vi "Control_demo.vi"(1 "stop":bool) -> (7 "liveview":dbl[][](graph))   [LabVIEW 2016]
uses:
  Vital supporting file for labview program/LV-EDSDK-Distribution_0.2/Distribution/EDSDK-Labview.llb/kEdsProperties.ctl
  Vital supporting file for labview program/LV-EDSDK-Distribution_0.2/Distribution/EDSDK-Labview.llb/kEdsCameraCommands.ctl
  Vital supporting file for labview program/C++/Dll for liveview/x64/Debug/Dll for liveview.dll
panel:
  in  "y 4":i16
  in  "y 3":i16
  in  "y 2":i16
  in  "y":i16
  in  "X":cluster{i32, i32}(slide)={0, 24101949} scale=0.0..1000.0
  out "new picture":picture
  in  "Zoom Factor":dbl=0.15
  in  "file name":string="m200test.bmp"
  in  "Path":path=path "C:/Users/Administrator/Desktop"
  out "saved image":picture
  out "output array 2":u32[][](array[numeric])
  out "error out":errorcluster
  in  "shutter":bool
  in  "Shutter speed":u16(ring) items=["1/8000"=160, "1/6400"=157, "1/6000"=156, "1/5000"=155, "1/4000"=152, "1/3200"=149, "1/3000"=148, "1/2500"=147, "1/2000"=144, "1/1600"=141, "1/1500"=140, "1/1250"=139, "1/100"=136, "1/800"=133, "1/640"=131, "1/500"=128, "1/400"=125, "1/320"=123, "1/250"=120, "1/200"=117, "1/160"=115, "1/125"=112, "1/100"=109, "1/80"=107, "1/60"=104, "1/50"=101, "1/40"=99, "1/30"=96, "1/25"=93, "1/8"=80, "1/6"=77, "1/5"=75, "1/4"=72, "0\"3"=69, "0\"4"=67, "0\"5"=64, "0\"6"=61, "0\"7"=60, "0\"8"=59, "1\""=56, "1\"3"=53, "1\"5"=52, "1\"6"=51, "2\""=48, "2\"5"=45, "3\""=44, "3\"2"=43, "4\""=40, "5\""=37, "6\""=35, "8\""=32, "10\""=29, "13\""=27, "15\""=24, "20\""=21, "25\""=19, "30\""=16]
  in  "ISO":u32(ring) items=["Auto"=0, "50"=64, "100"=72, "125"=75, "160"=77, "200"=80, "250"=83, "320"=85, "400"=88, "500"=91, "640"=93, "800"=96, "1000"=99, "1250"=101, "1600"=104, "2000"=107, "2500"=109, "3200"=112, "4000"=115, "5000"=117, "6400"=120, "8000"=123, "10000"=125, "12800"=128, "25600"=136, "51200"=144, "102400"=152, "204800"=160, "409600"=168]
  out "outDeviceInfo":T1
  in  "error in (no error)":errorcluster
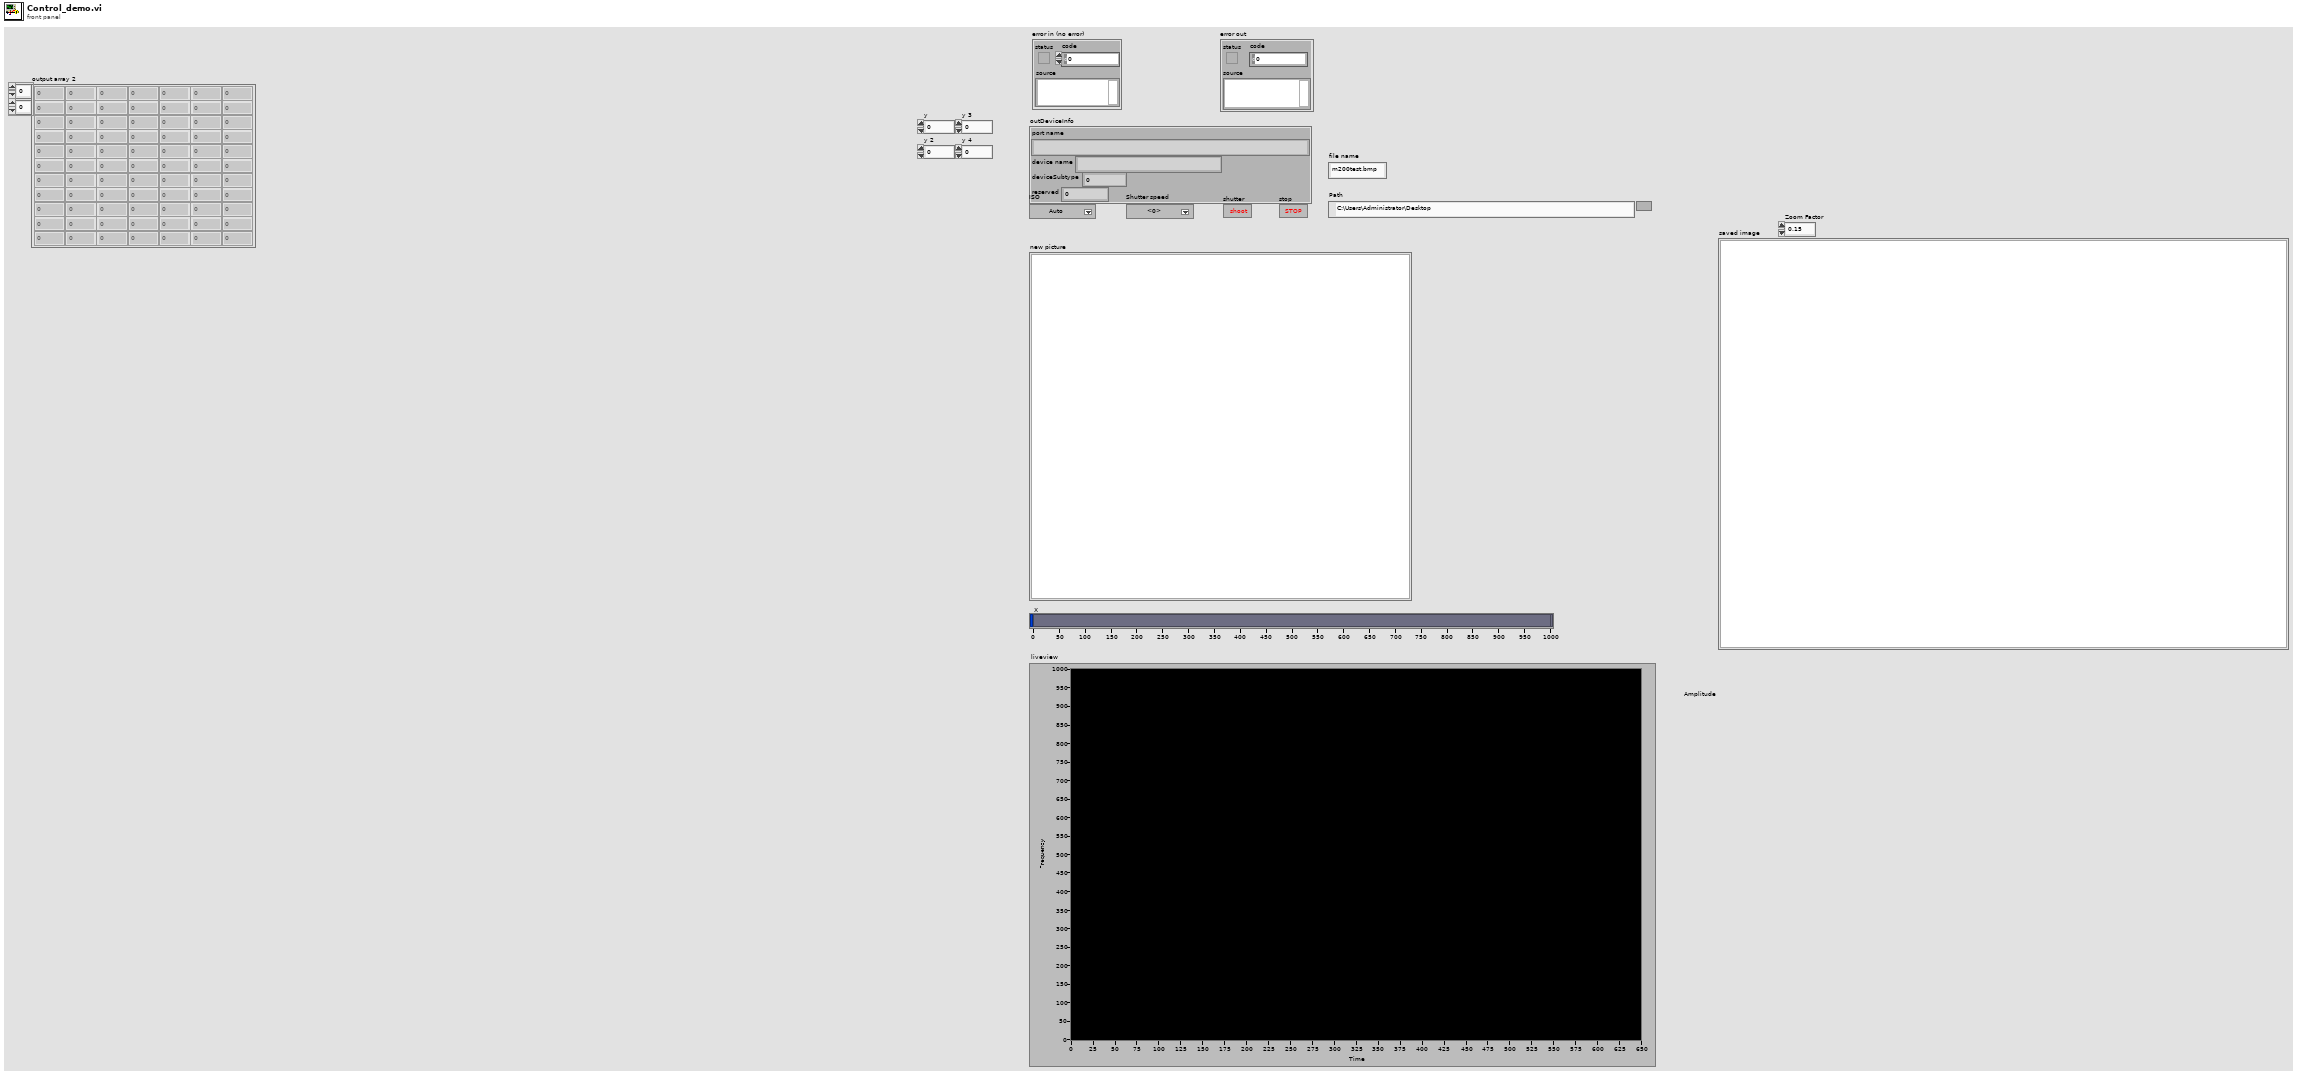
[diagram p1: front panel]
types:
  T1 = cluster{"port name":string, "device name":string, "deviceSubtype":u32, "reserved":u32}
  T2 = typedef "kEdsProperties.ctl" = u32
  T3 = enum16{"open", "replace", "create", "open or create", "replace or create", "replace or create with confirmation"}
  T4 = cluster{"Width":u16, "Style":enum32{"Solid", "Dash", "Dot", "DashDot", "DashDotDot"}}
  T5 = typedef "LVBoundsTypeDef.ctl" = cluster{"Width":u32, "Height":u32}
  T6 = typedef "imagedata.ctl" = cluster{"image type":i32, "image depth":i32, "image":u8[], "mask":u8[], "colors":u32[], "Rectangle":cluster{"left":i16, "top":i16, "right":i16, "bottom":i16}}
  T7 = cluster{"left":i16, "top":i16, "right":i16, "bottom":i16}
  T8 = typedef "kEdsCameraCommands.ctl" = u32
  T9 = typedef "LVMouseTypeDef.ctl" = cluster{"Mouse Position":cluster{"X":i32, "Y":i32}, "Mouse Modifiers":cluster{"Button Down":bool, "Shift Mod":bool, "Menu Mod":bool, "Option Mod":bool}}
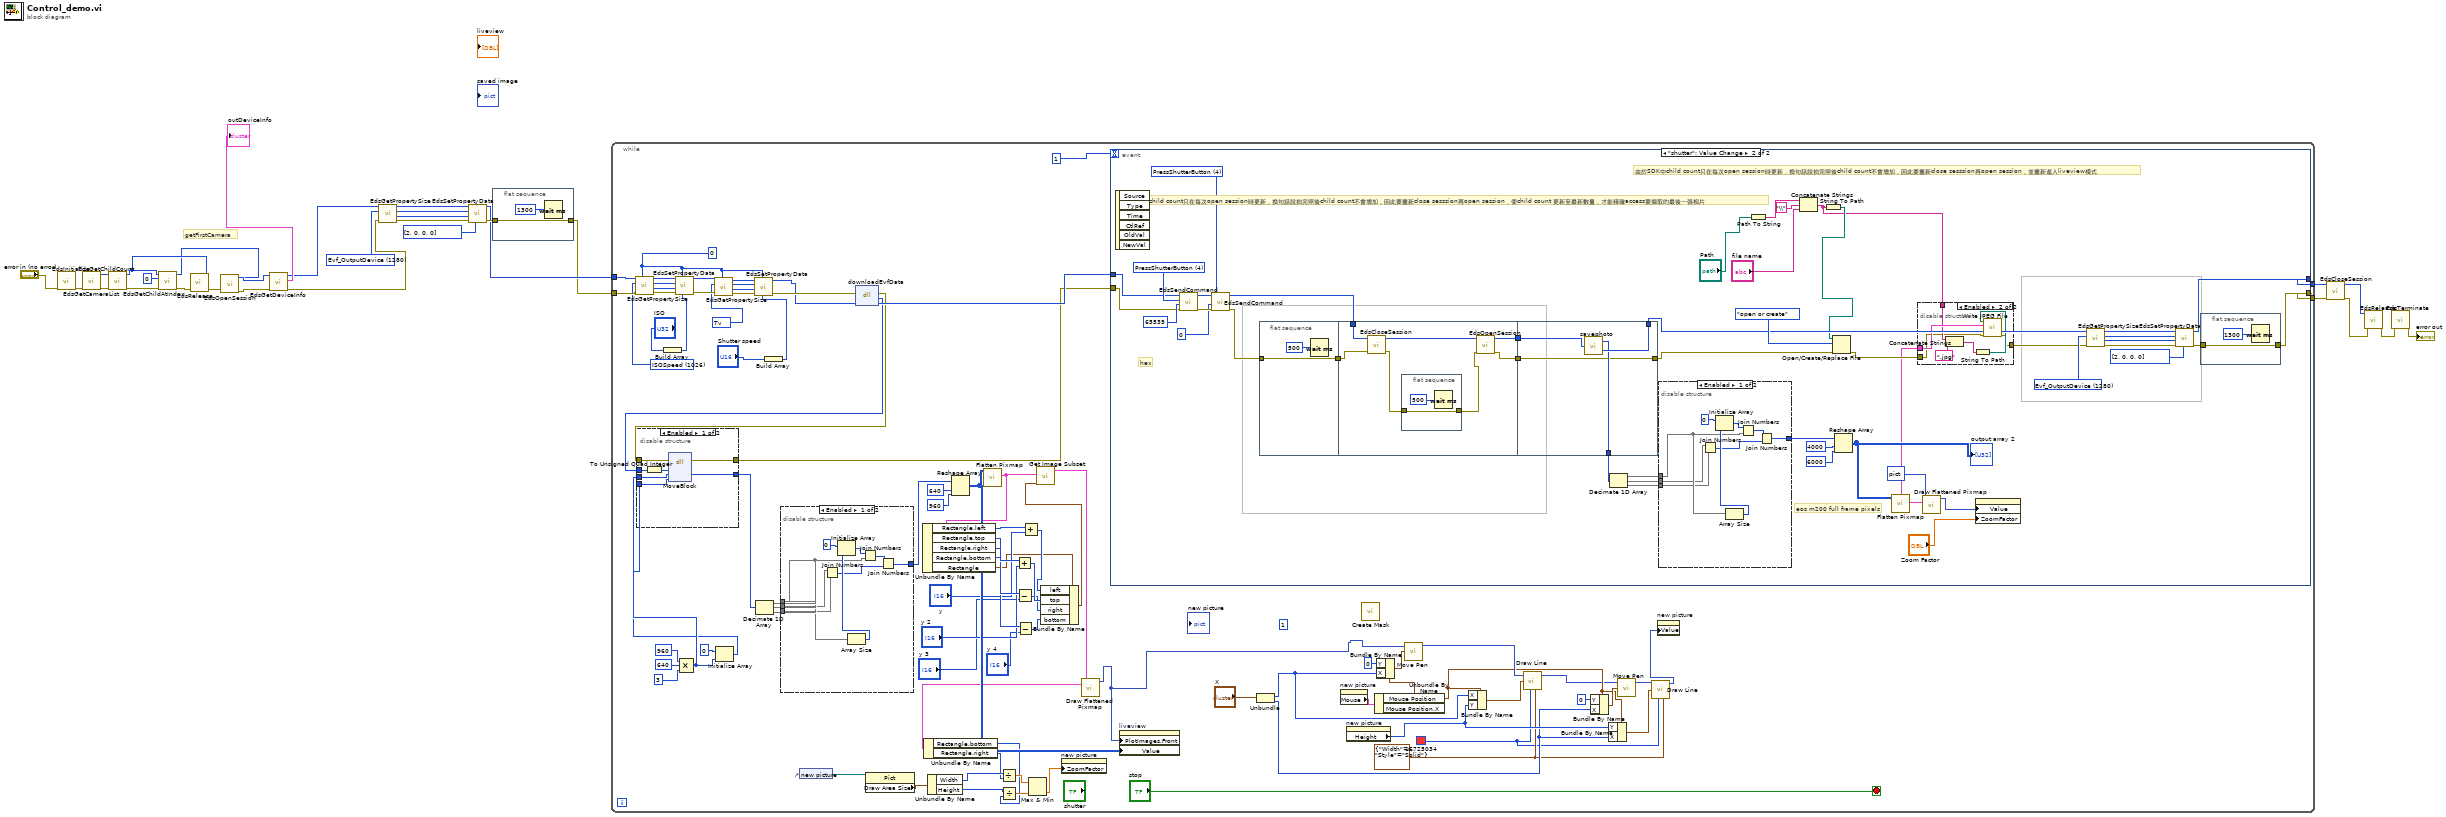
[diagram p0: block diagram]
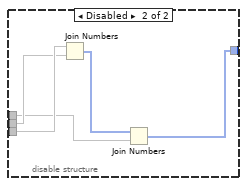
[diagram p2: hidden frame]
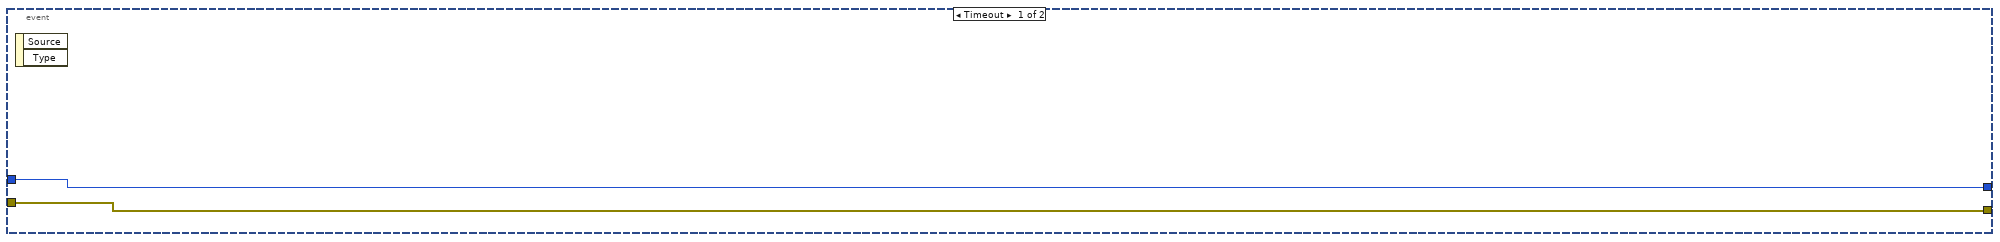
[diagram p4: hidden frame]
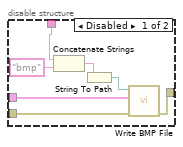
[diagram p5: hidden frame]
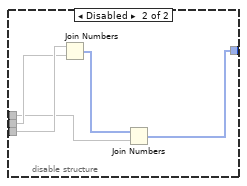
[diagram p6: hidden frame]
diagram:
  w5 = T2 1280 items=["Unknown"=65535, "ProductName"=2, "BodyID"=3, "OwnerName"=4, "MakerName"=5, "DateTime"=6, "FirmwareVersion"=7, "BatteryLevel"=8, "CFn"=9, "SaveTo"=11, "CurrentStorage"=12, "CurrentFolder"=13, "MyMenu"=14, "BatteryQuality"=16, "HDDirectoryStructure"=32, "ImageQuality"=256, "JpegQuality"=257, "Orientation"=258, "ICCProfile"=259, "FocusInfo"=260, "DigitalExposure"=261, "WhiteBalance"=262, "ColorTemperature"=263, "WhiteBalanceShift"=264, "Contrast"=265, "ColorSaturation"=266, "ColorTone"=267, "Sharpness"=268, "ColorSpace"=269, "ToneCurve"=270, "PhotoEffect"=271, "FilterEffect"=272, "ToningEffect"=273, "ParameterSet"=274, "ColorMatrix"=275, "PictureStyle"=276, "PictureStyleDesc"=277, "ETTL2Mode"=279, "PictureStyleCaption"=512, "Linear"=768, "ClickWBPoint"=769, "WBCoeffs"=770, "GPSVersionID"=2048, "GPSLatitudeRef"=2049, "GPSLatitude"=2050, "GPSLongitudeRef"=2051, "GPSLongitude"=2052, "GPSAltitudeRef"=2053, "GPSAltitude"=2054, "GPSTimeStamp"=2055, "GPSSatellites"=2056, "GPSStatus"=2057, "GPSMapDatum"=2066, "GPSDateStamp"=2077, "AtCapture_Flag"=2147483648, "AEMode"=1024, "DriveMode"=1025, "ISOSpeed"=1026, "MeteringMode"=1027, "AFMode"=1028, "Av"=1029, "Tv"=1030, "ExposureCompensation"=1031, "FlashCompensation"=1032, "FocalLength"=1033, "AvailableShots"=1034, "Bracket"=1035, "WhiteBalanceBracket"=1036, "LensName"=1037, "AEBracket"=1038, "FEBracket"=1039, "ISOBracket"=1040, "NoiseReduction"=1041, "FlashOn"=1042, "RedEye"=1043, "FlashMode"=1044, "LensStatus"=1046, "Artist"=1048, "Copyright"=1049, "DepthOfField"=1051, "EFCompensation"=1054, "Evf_OutputDevice"=1280, "Evf_Mode"=1281, "Evf_WhiteBalance"=1282, "Evf_ColorTemperature"=1283, "Evf_DepthOfFieldPreview"=1284, "Evf_Zoom"=1287, "Evf_ZoomPosition"=1288, "Evf_FocusAid"=1289, "Evf_Histogram"=1290, "Evf_ImagePosition"=1291, "Evf_HistogramStatus"=1292, "Evf_AFMode"=1294, "Evf_CoordinateSystem"=1344, "Evf_ZoomRect"=1345] ("inPropertyID")
  # "getFirstCamera"
  n1 = call "EdsInitialize.vi"("error in (no error)"="error in (no error)") -> ("error out"=w29:errorcluster)  [unwired: 10 in]
  n2 = call "EdsGetCameraList.vi"("error in"=w29) -> ("error out"=w28:errorcluster, "outCameraListRef"=w24:u32)  [unwired: 9 in]
  n3 = call "EdsGetChildCount.vi"("error in"=w28, "inRef"=w24) -> ("error out"=w27:errorcluster, "inRef dup"=w23:u32)  [unwired: 7 in, 1 out]
  n4 = call "EdsGetChildAtIndex.vi"("error in"=w27, "index"=u32 0, "inRef"=w23) -> ("error out"=w25:errorcluster, "outRef"=w19:u32)  [unwired: 7 in]
  n5 = call "EdsRelease.vi"("error in"=w25, "inRef"=w23) -> ("error out"=w22:errorcluster)  [unwired: 7 in, 2 out]
  n6 = call "EdsOpenSession.vi"("error in"=w22, "inCameraRef"=w19) -> ("error out"=w20:errorcluster, "inCameraRef dup"=w21:u32)  [unwired: 8 in]
  n7 = call "EdsGetDeviceInfo.vi"("error in"=w20, "inCameraRef"=w21) -> ("error out"=w2:errorcluster, "outDeviceInfo"=→"outDeviceInfo":T1, "inCameraRef dup"=w4:u32)  [unwired: 7 in]
  n8 = call "EdsGetPropertySize.vi"("error in"=w2, "inPropertyID"=w5, "inRef"=w4) -> ("error out"=w8:errorcluster, "outSize"=w9:u32, "inPropertyID dup"=w7:T2, "inRef dup"=w6:u32)  [unwired: 4 in, 1 out]
  n9 = call "EdsSetPropertyData.vi"("inPropertyData"=u8[] [2, 0, 0, 0], "error in"=w8, "inPropertySize"=w9, "inPropertyID"=w7, "inRef"=w6) -> ("error out"=w11:errorcluster, "inRef dup"=w3:u32)  [unwired: 5 in]
  n10 = flat-sequence {
    tunnel: w11 -> [w32]
    tunnel: [w32] -> w1
    frame #0 {
      n11 = Wait (ms)(milliseconds to wait=u32 1300) -> ()  [unwired: 1 out]
    }
  }
  n12 = while {
    tunnel: w3 -> [w100]
    tunnel: w1 -> [w119]
    tunnel: [w78] -> w13
    tunnel: [w79] -> w12
    stop <- "stop" stop-if-true
    w52 = T4 {"Width"=6, "Style"=enum."Solid"} ("pen")
    w51 = u32 16725034 ("color(black)")
    (unwired) 1
    w101 = T2 1030 items=["Unknown"=65535, "ProductName"=2, "BodyID"=3, "OwnerName"=4, "MakerName"=5, "DateTime"=6, "FirmwareVersion"=7, "BatteryLevel"=8, "CFn"=9, "SaveTo"=11, "CurrentStorage"=12, "CurrentFolder"=13, "MyMenu"=14, "BatteryQuality"=16, "HDDirectoryStructure"=32, "ImageQuality"=256, "JpegQuality"=257, "Orientation"=258, "ICCProfile"=259, "FocusInfo"=260, "DigitalExposure"=261, "WhiteBalance"=262, "ColorTemperature"=263, "WhiteBalanceShift"=264, "Contrast"=265, "ColorSaturation"=266, "ColorTone"=267, "Sharpness"=268, "ColorSpace"=269, "ToneCurve"=270, "PhotoEffect"=271, "FilterEffect"=272, "ToningEffect"=273, "ParameterSet"=274, "ColorMatrix"=275, "PictureStyle"=276, "PictureStyleDesc"=277, "ETTL2Mode"=279, "PictureStyleCaption"=512, "Linear"=768, "ClickWBPoint"=769, "WBCoeffs"=770, "GPSVersionID"=2048, "GPSLatitudeRef"=2049, "GPSLatitude"=2050, "GPSLongitudeRef"=2051, "GPSLongitude"=2052, "GPSAltitudeRef"=2053, "GPSAltitude"=2054, "GPSTimeStamp"=2055, "GPSSatellites"=2056, "GPSStatus"=2057, "GPSMapDatum"=2066, "GPSDateStamp"=2077, "AtCapture_Flag"=2147483648, "AEMode"=1024, "DriveMode"=1025, "ISOSpeed"=1026, "MeteringMode"=1027, "AFMode"=1028, "Av"=1029, "Tv"=1030, "ExposureCompensation"=1031, "FlashCompensation"=1032, "FocalLength"=1033, "AvailableShots"=1034, "Bracket"=1035, "WhiteBalanceBracket"=1036, "LensName"=1037, "AEBracket"=1038, "FEBracket"=1039, "ISOBracket"=1040, "NoiseReduction"=1041, "FlashOn"=1042, "RedEye"=1043, "FlashMode"=1044, "LensStatus"=1046, "Artist"=1048, "Copyright"=1049, "DepthOfField"=1051, "EFCompensation"=1054, "Evf_OutputDevice"=1280, "Evf_Mode"=1281, "Evf_WhiteBalance"=1282, "Evf_ColorTemperature"=1283, "Evf_DepthOfFieldPreview"=1284, "Evf_Zoom"=1287, "Evf_ZoomPosition"=1288, "Evf_FocusAid"=1289, "Evf_Histogram"=1290, "Evf_ImagePosition"=1291, "Evf_HistogramStatus"=1292, "Evf_AFMode"=1294, "Evf_CoordinateSystem"=1344, "Evf_ZoomRect"=1345] ("inPropertyID")
    w103 = 0 ("inParam")
    w113 = T2 1026 items=["Unknown"=65535, "ProductName"=2, "BodyID"=3, "OwnerName"=4, "MakerName"=5, "DateTime"=6, "FirmwareVersion"=7, "BatteryLevel"=8, "CFn"=9, "SaveTo"=11, "CurrentStorage"=12, "CurrentFolder"=13, "MyMenu"=14, "BatteryQuality"=16, "HDDirectoryStructure"=32, "ImageQuality"=256, "JpegQuality"=257, "Orientation"=258, "ICCProfile"=259, "FocusInfo"=260, "DigitalExposure"=261, "WhiteBalance"=262, "ColorTemperature"=263, "WhiteBalanceShift"=264, "Contrast"=265, "ColorSaturation"=266, "ColorTone"=267, "Sharpness"=268, "ColorSpace"=269, "ToneCurve"=270, "PhotoEffect"=271, "FilterEffect"=272, "ToningEffect"=273, "ParameterSet"=274, "ColorMatrix"=275, "PictureStyle"=276, "PictureStyleDesc"=277, "ETTL2Mode"=279, "PictureStyleCaption"=512, "Linear"=768, "ClickWBPoint"=769, "WBCoeffs"=770, "GPSVersionID"=2048, "GPSLatitudeRef"=2049, "GPSLatitude"=2050, "GPSLongitudeRef"=2051, "GPSLongitude"=2052, "GPSAltitudeRef"=2053, "GPSAltitude"=2054, "GPSTimeStamp"=2055, "GPSSatellites"=2056, "GPSStatus"=2057, "GPSMapDatum"=2066, "GPSDateStamp"=2077, "AtCapture_Flag"=2147483648, "AEMode"=1024, "DriveMode"=1025, "ISOSpeed"=1026, "MeteringMode"=1027, "AFMode"=1028, "Av"=1029, "Tv"=1030, "ExposureCompensation"=1031, "FlashCompensation"=1032, "FocalLength"=1033, "AvailableShots"=1034, "Bracket"=1035, "WhiteBalanceBracket"=1036, "LensName"=1037, "AEBracket"=1038, "FEBracket"=1039, "ISOBracket"=1040, "NoiseReduction"=1041, "FlashOn"=1042, "RedEye"=1043, "FlashMode"=1044, "LensStatus"=1046, "Artist"=1048, "Copyright"=1049, "DepthOfField"=1051, "EFCompensation"=1054, "Evf_OutputDevice"=1280, "Evf_Mode"=1281, "Evf_WhiteBalance"=1282, "Evf_ColorTemperature"=1283, "Evf_DepthOfFieldPreview"=1284, "Evf_Zoom"=1287, "Evf_ZoomPosition"=1288, "Evf_FocusAid"=1289, "Evf_Histogram"=1290, "Evf_ImagePosition"=1291, "Evf_HistogramStatus"=1292, "Evf_AFMode"=1294, "Evf_CoordinateSystem"=1344, "Evf_ZoomRect"=1345] ("inPropertyID")
    n13 = call "EdsGetPropertySize.vi"("inParam"=w103, "error in"=w119, "inPropertyID"=w113, "inRef"=w100) -> ("error out"=w115:errorcluster, "outSize"=w114:u32, "inPropertyID dup"=w116:T2, "inRef dup"=w117:u32)  [unwired: 3 in, 1 out]
    n14 = Build Array("ISO") -> (w111:u32[])
    n15 = call "EdsSetPropertyData.vi"("inPropertyData"=w111, "inParam"=w103, "error in"=w115, "inPropertySize"=w114, "inPropertyID"=w116, "inRef"=w117) -> ("error out"=w109:errorcluster, "inRef dup"=w102:u32)  [unwired: 4 in]
    n16 = Compound Arithmetic op=MULTIPLY(960 ("dimension size"), 640 ("dimension size"), 3 ("dimension size")) -> (w89:i32)
    n17 = call "EdsGetPropertySize.vi"("inParam"=w103, "error in"=w109, "inPropertyID"=w101, "inRef"=w102) -> ("error out"=w108:errorcluster, "outSize"=w106:u32, "inPropertyID dup"=w110:T2, "inRef dup"=w107:u32)  [unwired: 3 in, 1 out]
    n18 = Initialize Array ("初始化数组")(u8 0 ("element"), w89) -> (w88:u8[])
    n19 = Build Array("Shutter speed") -> (w104:u16[])
    n20 = call "EdsSetPropertyData.vi"("inPropertyData"=w104, "inParam"=w103, "error in"=w108, "inPropertySize"=w106, "inPropertyID"=w110, "inRef"=w107) -> ("error out"=w99:errorcluster, "inRef dup"=w98:u32)  [unwired: 4 in]
    n21 = control-ref of="new picture"() -> (w68:refnum<vi>)
    n22 = dll-call lib="D:/All users/PoSheng/src/labview for canon om/Vital supporting file for labview program/C++/Dll for liveview/x64/Debug/Dll for liveview.dll" fn="downloadEvfData"(error in=w99, "CamRef"=w98) -> (error out=w83:errorcluster, "return type"=w81:i64, "CamRef"=w97:u32)  [unwired: 2 in, 1 out]
    n23 = disable-structure shown="Enabled" {
      disable-tunnel: [w140 w141] -> w82
      disable-tunnel: w81 -> [w139 _]
      disable-tunnel: w83 -> [w138 w141]
      disable-tunnel: w88 -> [w137 _]
      disable-tunnel: w89 -> [w136 _]
      disable-tunnel: [w134 _] -> w96
      frame Enabled {
        n24 = To Unsigned Quad Integer(1:w139) -> (0:w135:u64)
        n25 = dll-call lib="LabVIEW" fn="MoveBlock"(error in=w138, "src"=w135, "dst"=w137, "size"=w136) -> (error out=w140:errorcluster, "dst"=w134:u8[])  [unwired: 5 in, 1 out]
      }
      frame Disabled {
      }
    }
    n26 = Decimate 1D Array(w96) -> (w91:u8[], w90:u8[], w92:u8[])
    n27 = disable-structure shown="Enabled" {
      disable-tunnel: w90 -> [w121 w130]
      disable-tunnel: w91 -> [w122 w129]
      disable-tunnel: w92 -> [w120 w131]
      disable-tunnel: [w123 w132] -> w93
      frame Enabled {
        n28 = Join Numbers(hi=w121, lo=w120) -> ((hi.lo)=w124:u16[])
        n29 = Array Size(array=w122) -> (size(s)=w127:i32)
        n30 = Initialize Array(u8 0, w127) -> (w126:u8[])
        n31 = Join Numbers(hi=w126, lo=w122) -> ((hi.lo)=w125:u16[])
        n32 = Join Numbers(hi=w125, lo=w124) -> ((hi.lo)=w123:u32[])
      }
      frame Disabled {
        n33 = Join Numbers(hi=w131, lo=w130) -> ((hi.lo)=w133:u16[])
        n34 = Join Numbers(hi=w133, lo=w129) -> ((hi.lo)=w132:u32[])
      }
    }
    n35 = property on="Property Node" class="Pict"(reference=w68) -> ("Draw Area Size"=w76:T5)  [unwired: 1 in, 2 out]
    n36 = Unbundle By Name(w76) -> ("Width"=w75:u32, "Height"=w73:u32)
    n37 = Reshape Array(w93, 640 ("dimension size"), 960 ("dimension size")) -> (w80:u32[][])
    n38 = call <vilib>:"Flatten Pixmap.vi"("24-bit pixmap"=w80) -> ("image data"=w47:T6)  [unwired: 10 in]
    n39 = Unbundle By Name(w47) -> ("Rectangle.left"=w46:i16, "Rectangle.top"=w45:i16, "Rectangle.right"=w44:i16, "Rectangle.bottom"=w43:i16, "Rectangle"=w37:T7)
    n40 = Add(x=w45, y="y 2") -> (x+y=w35:i16)
    n41 = Subtract(x=w44, y="y 3") -> (x-y=w34:i16)
    n42 = Subtract(x=w43, y="y 4") -> (x-y=w33:i16)
    n43 = Add(x=w46, y="y") -> (x+y=w38:i16)
    n44 = Bundle By Name(cluster=w37, "left"=w38, "top"=w35, "right"=w34, "bottom"=w33) -> (w36:T7)
    n45 = call <vilib>:"Get Image Subset.vi"("subset rect"=w36, "image data"=w47) -> ("image subset"=w48:T6)  [unwired: 4 in, 1 out]
    n46 = Unbundle By Name(w48) -> ("Rectangle.bottom"=w70:i16, "Rectangle.right"=w74:i16)
    n47 = Divide(x=w75, y=w74) -> (x/y=w72:dbl)
    n48 = Divide(x=w73, y=w70) -> (x/y=w71:dbl)
    n49 = Max & Min(x=w72, y=w71) -> (min(x,y)=w69:dbl)  [unwired: 1 out]
    n50 = property on="new picture" class="Pict"("ZoomFactor"=w69) -> ()  [unwired: 2 in, 2 out]
    n51 = call <vilib>:"Draw Flattened Pixmap.vi"("image data"=w48) -> ("new picture"=w62:picture)  [unwired: 8 in]
    n52 = event shown="[1] \"shutter\": Value Change" {
      selector: _ -> [_ _]
      dyn-events: _ -> [_ _]
      timeout: 1 -> [_ _]
      tunnel: [w142 w158] -> w78
      tunnel: [w143 w153] -> w79
      tunnel: w97 -> [w143 w182]
      tunnel: w82 -> [w142 w181]
      event Timeout {
        n53 = event-data() -> ()  [unwired: 1 in, 2 out]
      }
      event "shutter": Value Change {
        w165 = T2 1280 items=["Unknown"=65535, "ProductName"=2, "BodyID"=3, "OwnerName"=4, "MakerName"=5, "DateTime"=6, "FirmwareVersion"=7, "BatteryLevel"=8, "CFn"=9, "SaveTo"=11, "CurrentStorage"=12, "CurrentFolder"=13, "MyMenu"=14, "BatteryQuality"=16, "HDDirectoryStructure"=32, "ImageQuality"=256, "JpegQuality"=257, "Orientation"=258, "ICCProfile"=259, "FocusInfo"=260, "DigitalExposure"=261, "WhiteBalance"=262, "ColorTemperature"=263, "WhiteBalanceShift"=264, "Contrast"=265, "ColorSaturation"=266, "ColorTone"=267, "Sharpness"=268, "ColorSpace"=269, "ToneCurve"=270, "PhotoEffect"=271, "FilterEffect"=272, "ToningEffect"=273, "ParameterSet"=274, "ColorMatrix"=275, "PictureStyle"=276, "PictureStyleDesc"=277, "ETTL2Mode"=279, "PictureStyleCaption"=512, "Linear"=768, "ClickWBPoint"=769, "WBCoeffs"=770, "GPSVersionID"=2048, "GPSLatitudeRef"=2049, "GPSLatitude"=2050, "GPSLongitudeRef"=2051, "GPSLongitude"=2052, "GPSAltitudeRef"=2053, "GPSAltitude"=2054, "GPSTimeStamp"=2055, "GPSSatellites"=2056, "GPSStatus"=2057, "GPSMapDatum"=2066, "GPSDateStamp"=2077, "AtCapture_Flag"=2147483648, "AEMode"=1024, "DriveMode"=1025, "ISOSpeed"=1026, "MeteringMode"=1027, "AFMode"=1028, "Av"=1029, "Tv"=1030, "ExposureCompensation"=1031, "FlashCompensation"=1032, "FocalLength"=1033, "AvailableShots"=1034, "Bracket"=1035, "WhiteBalanceBracket"=1036, "LensName"=1037, "AEBracket"=1038, "FEBracket"=1039, "ISOBracket"=1040, "NoiseReduction"=1041, "FlashOn"=1042, "RedEye"=1043, "FlashMode"=1044, "LensStatus"=1046, "Artist"=1048, "Copyright"=1049, "DepthOfField"=1051, "EFCompensation"=1054, "Evf_OutputDevice"=1280, "Evf_Mode"=1281, "Evf_WhiteBalance"=1282, "Evf_ColorTemperature"=1283, "Evf_DepthOfFieldPreview"=1284, "Evf_Zoom"=1287, "Evf_ZoomPosition"=1288, "Evf_FocusAid"=1289, "Evf_Histogram"=1290, "Evf_ImagePosition"=1291, "Evf_HistogramStatus"=1292, "Evf_AFMode"=1294, "Evf_CoordinateSystem"=1344, "Evf_ZoomRect"=1345] ("inPropertyID")
        w184 = T8 4 items=["TakePicture"=0, "ExtendShutDownTimer"=1, "BulbStart"=2, "BulbEnd"=3, "DoEvfAf"=258, "DriveLensEvf"=259, "DoClickWBEvf"=260, "PressShutterButton"=4] ("inCommand")
        w188 = T8 4 items=["TakePicture"=0, "ExtendShutDownTimer"=1, "BulbStart"=2, "BulbEnd"=3, "DoEvfAf"=258, "DriveLensEvf"=259, "DoClickWBEvf"=260, "PressShutterButton"=4] ("inCommand")
        # "eos m200 full frame pixels"
        # "hex"
        # "由於SDK中child count只在每次open session時更新，換句話說拍完照後child count不會增加，因此要重新close sesssion再open session，並重新進入liveview模式"
        # "由於SDK中child count只在每次open session時更新，換句話說拍完照後child count不會增加，因此要重新close sesssion再open session，使child count 更新至最新數量，才能精確access要擷取的最後一張相片"
        n54 = event-data() -> ()  [unwired: 1 in, 6 out]
        n55 = call "EdsSendCommand.vi"("error in"=w181, "inParam"=65539, "inCommand"=w188, "inRef"=w182) -> ("error out"=w186:errorcluster, "inRef dup"=w185:u32)  [unwired: 2 in]
        n56 = call "EdsSendCommand.vi"("error in"=w186, "inParam"=0, "inCommand"=w184, "inRef"=w185) -> ("error out"=w169:errorcluster, "inRef dup"=w152:u32)  [unwired: 2 in]
        n57 = flat-sequence {
          tunnel: w169 -> [w206]
          tunnel: [w206] -> w157
          tunnel: w157 -> [w210]
          tunnel: [w209] -> w156
          tunnel: w152 -> [w208]
          tunnel: [w207] -> w151
          tunnel: [w217] -> w166
          tunnel: w156 -> [w217]
          tunnel: [w219] -> w154
          tunnel: [w218] -> w167
          tunnel: w151 -> [w216]
          frame #0 {
            n58 = Wait (ms)(milliseconds to wait=u32 500) -> ()  [unwired: 1 out]
          }
          frame #1 {
            n59 = call "EdsCloseSession.vi"("error in"=w210, "inCameraRef"=w208) -> ("error out"=w212:errorcluster, "inCameraRef dup"=w211:u32)  [unwired: 8 in]
            n60 = flat-sequence {
              tunnel: w212 -> [w215]
              tunnel: [w215] -> w213
              frame #0 {
                n61 = Wait (ms)(milliseconds to wait=u32 500) -> ()  [unwired: 1 out]
              }
            }
            n62 = call "EdsOpenSession.vi"("error in"=w213, "inCameraRef"=w211) -> ("error out"=w209:errorcluster, "inCameraRef dup"=w207:u32)  [unwired: 8 in]
          }
          frame #2 {
            n63 = call "savephoto.vi"("camera"=w216) -> ("dst"=w218:u8[], "camera 2"=w219:u32)
          }
        }
        n64 = Decimate 1D Array(w167) -> (w177:u8[], w178:u8[], w176:u8[])
        n65 = disable-structure shown="Enabled" {
          disable-tunnel: w178 -> [w221 w230]
          disable-tunnel: w177 -> [w222 w229]
          disable-tunnel: w176 -> [w220 w231]
          disable-tunnel: [w223 w232] -> w175
          frame Enabled {
            n66 = Join Numbers(hi=w221, lo=w220) -> ((hi.lo)=w224:u16[])
            n67 = Array Size(array=w222) -> (size(s)=w227:i32)
            n68 = Initialize Array(u8 0, w227) -> (w226:u8[])
            n69 = Join Numbers(hi=w226, lo=w222) -> ((hi.lo)=w225:u16[])
            n70 = Join Numbers(hi=w225, lo=w224) -> ((hi.lo)=w223:u32[])
          }
          frame Disabled {
            n71 = Join Numbers(hi=w231, lo=w230) -> ((hi.lo)=w233:u16[])
            n72 = Join Numbers(hi=w233, lo=w229) -> ((hi.lo)=w232:u32[])
          }
        }
        n73 = Path To String(path="Path") -> (string=w149:string)
        n74 = Concatenate Strings(w149, "\\", "file name") -> (w144:string)
        n75 = String To Path(string=w144) -> (path=w146:path)
        n76 = Open/Create/Replace File(file path (use dialog)=w146, error in=w166, operation (0:open)=T3."open or create") -> (error out=w170:errorcluster)  [unwired: 3 in, 2 out]
        n77 = Reshape Array(w175, 4000 ("dimension size"), 6000 ("dimension size")) -> (w180:u32[][])
        "output array 2" <- w180
        n78 = call <vilib>:"Flatten Pixmap.vi"("24-bit pixmap"=w180) -> ("image data"=w145:T6)  [unwired: 10 in]
        n79 = disable-structure shown="Enabled" {
          disable-tunnel: w170 -> [w195 w197]
          disable-tunnel: [w194 w196] -> w155
          disable-tunnel: w145 -> [w193 w200]
          disable-tunnel: w144 -> [w192 w199]
          frame Disabled {
            n80 = Concatenate Strings(w192, "bmp" ("string")) -> (w190:string)
            n81 = String To Path(string=w190) -> (path=w189:path)
            n82 = call <vilib>:"Write BMP File.vi"("error in (no error)"=w195, "image data"=w193, "path to BMP file"=w189) -> ("error out"=w194:errorcluster)  [unwired: 7 in, 1 out]
          }
          frame Enabled {
            n83 = Concatenate Strings(w199, ".jpg" ("string")) -> (w202:string)
            n84 = String To Path(string=w202) -> (path=w198:path)
            n85 = call <vilib>:"Write JPEG File.vi"("error in (no error)"=w197, "image data"=w200, "path to JPEG file"=w198) -> ("error out"=w196:errorcluster)  [unwired: 7 in, 1 out]
          }
        }
        n86 = call <vilib>:"Draw Flattened Pixmap.vi"("image data"=w145, "picture"=picture data[5B]) -> ("new picture"=w172:picture)  [unwired: 7 in]
        n87 = property on="saved image" class="Pict"("Value"=w172, "ZoomFactor"="Zoom Factor") -> ()  [unwired: 2 in, 2 out]
        n88 = call "EdsGetPropertySize.vi"("error in"=w155, "inPropertyID"=w165, "inRef"=w154) -> ("error out"=w162:errorcluster, "outSize"=w161:u32, "inPropertyID dup"=w163:T2, "inRef dup"=w164:u32)  [unwired: 4 in, 1 out]
        n89 = call "EdsSetPropertyData.vi"("inPropertyData"=u8[] [2, 0, 0, 0], "error in"=w162, "inPropertySize"=w161, "inPropertyID"=w163, "inRef"=w164) -> ("error out"=w159:errorcluster, "inRef dup"=w153:u32)  [unwired: 5 in]
        n90 = flat-sequence {
          tunnel: w159 -> [w204]
          tunnel: [w204] -> w158
          frame #0 {
            n91 = Wait (ms)(milliseconds to wait=u32 1300) -> ()  [unwired: 1 out]
          }
        }
      }
    }
    n92 = property on="liveview" class="IntGraph (strict)"("PlotImages.Front"=w62, "Value"=w80) -> ()  [unwired: 2 in, 2 out]
    n93 = Unbundle("X") -> (w60:i32, w53:i32)
    n94 = property on="new picture" class="Pict"() -> ("Mouse"=w67:T9)  [unwired: 2 in, 2 out]
    n95 = property on="new picture" class="Pict"() -> ("Height"=w54:u32)  [unwired: 2 in, 2 out]
    n96 = call <vilib>:"Create Mask.vi"() -> ()  [unwired: 11 in, 1 out]
    n97 = Unbundle By Name(w67) -> ("Mouse Position"=w56:cluster{"X":i32, "Y":i32})  [unwired: 1 out]
    n98 = Bundle By Name(cluster=w56, "Y"=0, "X"=w60) -> (w64:cluster{"X":i32, "Y":i32})
    n99 = call <vilib>:"Move Pen.vi"("new position"=w64, "picture"=w62) -> ("new picture"=w66:picture)  [unwired: 3 in]
    n100 = Bundle By Name(cluster=w56, "X"=w60, "Y"=w54) -> (w63:cluster{"X":i32, "Y":i32})
    n101 = call <vilib>:"Draw Line.vi"("picture"=w66, "end point"=w63, "color(black)"=w51, "pen"=w52) -> ("new picture"=w50:picture)  [unwired: 5 in]
    n102 = Bundle By Name(cluster=w56, "Y"=0, "X"=w53) -> (w58:cluster{"X":i32, "Y":i32})
    n103 = Bundle By Name(cluster=w56, "Y"=w54, "X"=w53) -> (w55:cluster{"X":i32, "Y":i32})
    n104 = call <vilib>:"Move Pen.vi"("new position"=w58, "picture"=w50) -> ("new picture"=w57:picture)  [unwired: 3 in]
    n105 = call <vilib>:"Draw Line.vi"("picture"=w57, "end point"=w55, "color(black)"=w51, "pen"=w52) -> ("new picture"=w49:picture)  [unwired: 5 in]
    n106 = property on="new picture" class="Pict"("Value"=w49) -> ()  [unwired: 2 in, 2 out]
  }
  n107 = call "EdsCloseSession.vi"("error in"=w13, "inCameraRef"=w12) -> ("error out"=w17:errorcluster, "inCameraRef dup"=w14:u32)  [unwired: 8 in]
  n108 = call "EdsRelease.vi"("error in"=w17, "inRef"=w14) -> ("error out"=w15:errorcluster)  [unwired: 7 in, 2 out]
  n109 = call "EdsTerminate.vi"("error in"=w15) -> ("error out"=→"error out":errorcluster)  [unwired: 10 in]
